vi "LINXx - Switch to WiFi.vi"() -> ()   [LabVIEW 2019]
uses:
  <vilib>/MakerHub/LINX/Private/Type Defs/Interface.ctl
  <vilib>/MakerHub/LINX/Private/Device/Type Defs/Wifi Config.ctl
  <vilib>/MakerHub/LINX/Private/Type Defs/WIFI Security Type.ctl
  vi.lib/LINXx/Private/WiFi101 Status.ctl
  <vilib>/MakerHub/LINX/Public/Utilities/Open Serial.vi
  <vilib>/MakerHub/LINX/LMH-LINX.lvlib
  <vilib>/MakerHub/LINX/Private/Device/Device.lvlib
  vi.lib/LINXx/LINXx.lvlib
panel:
  in  "Switch wait time [ms]":u32=1000
  in  "WiFi retry wait time [ms]":u32=500
  in  "Board reset wait [ms]":u32=1000
  in  "Reset Board":bool
  in  "Reset WiFI":bool
  in  "stop":bool
  in  "Switch to WiFi connection":bool
  out "Loop Rate (Hz)":u32
  out "Connection":bool
  out "WiFi Status":T1 items=["No module"=255, "Idle"=0, "No SSID"=1, "Scan completed"=2, "Connected"=3, "Connection failed"=4, "Connection lost"=5, "Disconnected"=6, "AP listening"=7, "AP connected"=8, "AP failed"=9, "Provisioning"=10, "Provisioning failed"=11]
  in  "New Wifi Config":T2={"SSID"="", "IP Address"="", "Port"=0, "WIFI Security Type"=enum."WPA2 Password", "Password"=""}
  in  "Set WiFi info":bool
  out "Saved Wifi Configuration":T2={"SSID"="", "IP Address"="", "Port"=0, "WIFI Security Type"=enum."WPA2 Password", "Password"=""}
  in  "Get WiFi info":bool
  out "Current connection":T4
  in  "Serial Port":refnum<visa-resource-name>="N/A"
  # "Setup"
  # "Start with a serial connection to the LINX board.\nIf the network information was programmed in the firmware sketch,\nyou can get the saved values but changing them here has no effect.\nOtherwise, you can reconfigure & test new settings that will be saved across\nreboots.\nIf WiFi connection fails after new settings, try running the VI again."
  # "Status"
  # "Commands"
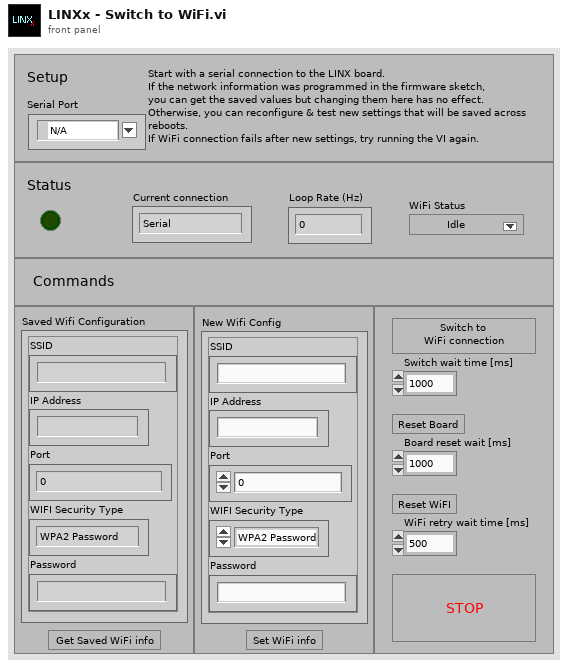
[diagram p1: front panel]
types:
  T1 = typedef "LINXx.lvlib/WiFi101 Status.ctl" = u8
  T2 = typedef "LMH-LINX.lvlib/Device.lvlib/Wifi Config.ctl" = cluster{"SSID":string, "IP Address":string, "Port":u16, "WIFI Security Type":T3, "Password":string}
  T3 = typedef "LMH-LINX.lvlib/WIFI Security Type.ctl" = enum8{"None", "WPA2 Password", "WPA2 Key", "WEP40", "WEP104"}
  T4 = typedef "LMH-LINX.lvlib/Interface.ctl" = enum16{"Serial", "TCP"}
  T5 = typedef "LMH-LINX.lvlib/LINX Ref.ctl" = cluster{"IO":T6, "Interface":T4, "LINX Device Config":T7}
  T6 = typedef "LMH-LINX.lvlib/Platform.ctl" = enum16{"Remote", "Local"}
  T7 = typedef "LMH-LINX.lvlib/Device.lvlib/LINX Device Config.ctl" = cluster{"Interface":T4, "COM Port":refnum<visa-resource-name>, "TCP Configuration":T8, "Device Family":u8, "Device ID":u8, "Device Name":string, "TCP Ref":refnum<k5>, "Channels":T9}
  T8 = typedef "LMH-LINX.lvlib/Device.lvlib/TCP Config.ctl" = cluster{"IP Address":string, "Port":u16}
  T9 = typedef "LMH-LINX.lvlib/Channels.ctl" = cluster{"DI":u8[], "DO":u8[], "AI":u8[], "AO":u8[], "PWM":u8[], "QE":u8[], "UART":u8[], "I2C 2":u8[], "SPI":u8[], "CAN":u8[], "Servo":u8[], "AI Ref (V)":dbl, "AI Resolution (Bits)":u8, "AO Ref (V)":dbl, "AO Resolution (Bits)":u8}
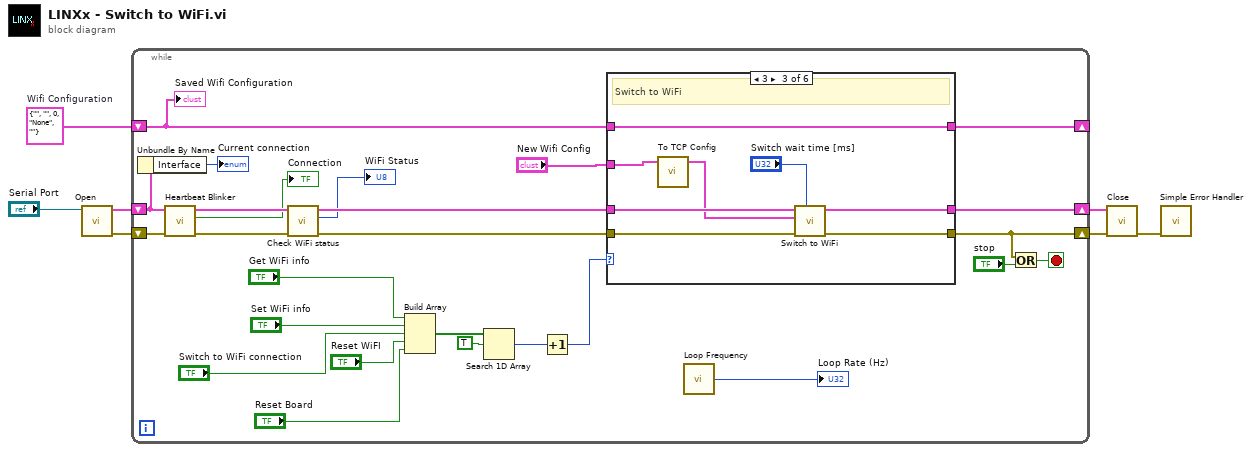
[diagram p0: block diagram]
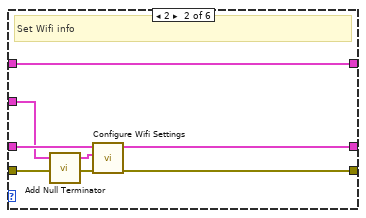
[diagram p3: hidden frame]
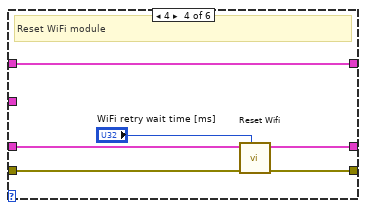
[diagram p4: hidden frame]
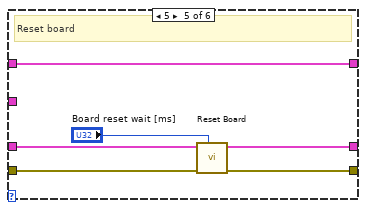
[diagram p5: hidden frame]
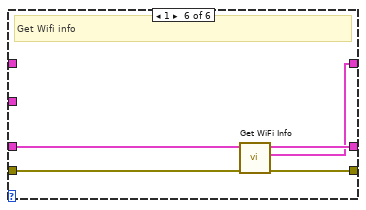
[diagram p6: hidden frame]
diagram:
  w4 = T2 {"SSID"="", "IP Address"="", "Port"=0, "WIFI Security Type"=enum."None", "Password"=""}  # Wifi Configuration
  n1 = call-poly <vilib>:"Open.vi"("Serial Port"="Serial Port") -> ("Error Out"=w5:errorcluster, "LINX Resource"=w6:T5)  [unwired: 8 in, 1 out]
  n2 = while {
    shift-right: [w21] -> w2
    shift-left: w6 -> [w9]
    shift-right: [w20] -> w3
    shift-left: w5 -> [w14]
    shift-right: [w31] -> _
    shift-left: w4 -> [w32]
    stop <- w22 stop-if-true
    n3 = Unbundle By Name(w9) -> ("Interface"=→"Current connection":T4)
    n4 = call "Heartbeat Blinker.vi"("Error In"=w14, "LINX Resource"=w9) -> ("Error Out"=w13:errorcluster, "LED"=→"Connection":bool, "LINX Resource Out"=w12:T5)  [unwired: 7 in]
    n5 = call "Check WiFi status.vi"("Error In"=w13, "LINX Resource"=w12) -> ("Error Out"=w17:errorcluster, "WiFi status"=→"WiFi Status":u8, "LINX Resource out"=w19:T5)  [unwired: 7 in]
    n6 = Build Array("Get WiFi info", "Set WiFi info", "Switch to WiFi connection", "Reset WiFI", "Reset Board") -> (w27:bool[])
    n7 = Search 1D Array(1D array=w27, element=TRUE) -> (index of element=w25:i32)  [unwired: 1 in]
    n8 = Increment(x=w25) -> (x+1=w24:i32)
    n9 = case shown="3" w24 {
      tunnel: w32 -> [w36 w39 w44 w57 w63 _]
      tunnel: [w36 w39 w44 w57 w63 w64] -> w31
      tunnel: w17 -> [w35 w43 w49 w55 w61 w68]
      tunnel: [w35 w42 w50 w54 w60 w67] -> w20
      tunnel: w19 -> [w34 w41 w48 w56 w62 w66]
      tunnel: [w34 w40 w51 w53 w59 w65] -> w21
      tunnel: "New Wifi Config" -> [_ w38 w45 _ _ _]
      frame 0, Default {
        # "idle"
      }
      frame 2 {
        # "Set Wifi info"
        n10 = call "Add Null Terminator.vi"("New Wifi Config in"=w38) -> ("New Wifi Config out"=w37:T2)  [unwired: 4 in]
        n11 = call <vilib>:"Configure Wifi Settings.vi"("Error In"=w43, "Wifi Configuration"=w37, "LINX Resource"=w41) -> ("Error Out"=w42:errorcluster, "LINX Resource"=w40:T5)  [unwired: 7 in]
      }
      frame 3 {
        # "Switch to WiFi"
        n12 = call "To TCP Config.vi"("Wifi Configuration"=w45) -> ("TCP Configuration"=w46:T8)  [unwired: 4 in]
        n13 = call "Switch to WiFi.vi"("Retry wait time [ms]"="Switch wait time [ms]", "Error In"=w49, "TCP Configuration"=w46, "LINX Resource"=w48) -> ("Error Out"=w50:errorcluster, "LINX Resource out"=w51:T5)  [unwired: 6 in]
      }
      frame 4 {
        # "Reset WiFi module"
        n14 = call "Reset Wifi.vi"("Retry wait time [ms]"="WiFi retry wait time [ms]", "error in (no error)"=w55, "LINX Resource"=w56) -> ("error out"=w54:errorcluster, "LINX Resource Out"=w53:T5)  [unwired: 5 in, 2 out]
      }
      frame 5 {
        # "Reset board"
        n15 = call "Reset Board.vi"("Reconnect wait time"="Board reset wait [ms]", "Error In"=w61, "LINX Resource"=w62) -> ("Error Out"=w60:errorcluster, "LINX Resource out"=w59:T5)  [unwired: 7 in]
      }
      frame 1 {
        # "Get Wifi info"
        n16 = call "Get WiFi Info.vi"("Error In"=w68, "LINX Resource"=w66) -> ("Error Out"=w67:errorcluster, "WiFi Info"=w64:T2, "LINX Resource Out"=w65:T5)  [unwired: 6 in, 1 out]
      }
    }
    n17 = call <vilib>:"Loop Frequency.vi"() -> ("Loop Rate (Hz)"=→"Loop Rate (Hz)":u32)
    n18 = Or(x=w20, y="stop") -> (x .or. y?=w22:bool)
    "Saved Wifi Configuration" <- w32
  }
  n19 = call <vilib>:"Close.vi"("Error In"=w3, "LINX Resource"=w2) -> ("Error Out"=w1:errorcluster)  [unwired: 9 in]
  n20 = call <vilib>:"Simple Error Handler.vi"("error in (no error)"=w1) -> ()  [unwired: 4 in, 5 out]
